vi "GetFill.vi"(8 "error in (no error)":errorcluster, 11 "Polygone in":refnum<class "Polygone.lvclass">) -> (0 "error out":errorcluster, 2 "Fill":bool, 3 "Polygone out":refnum<class "Polygone.lvclass">)   [LabVIEW 2021, in "Picture2D.lvlib" / "Polygone.lvclass"]
uses:
  Polygone.lvclass
  Polygone.lvclass/Polygone.ctl
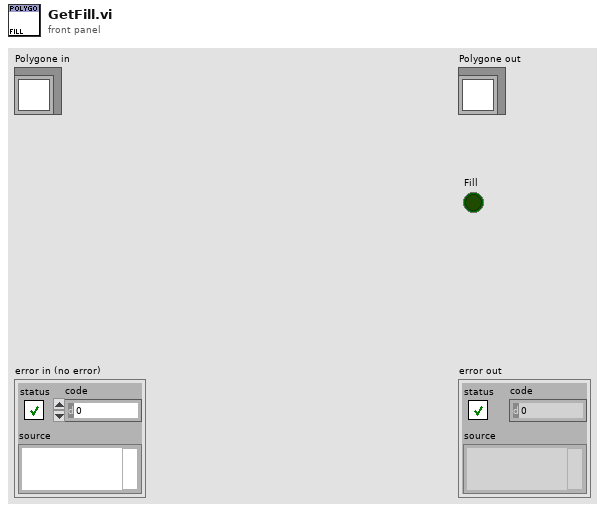
[diagram p1: front panel]
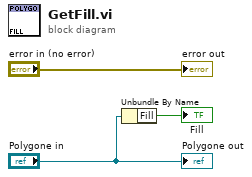
[diagram p0: block diagram]
diagram:
  n1 = Unbundle By Name("Polygone in") -> ("Fill"=→"Fill":bool)
  "error out" <- "error in (no error)"
  "Polygone out" <- "Polygone in"
